vi "GetFrontPanel.vi"(8 "Error In":errorcluster, 11 "object in":refnum<class "FooterTriekselSoft.lvclass">) -> (0 "Error Out":errorcluster, 2 "FrontPanel":refnum<class "FrontPanelControl.lvclass">, 3 "object out":refnum<class "FooterTriekselSoft.lvclass">)   [LabVIEW 2021, in "FooterTriekselSoft.lvclass"]
uses:
  FooterTriekselSoft.lvclass
  .Externals/Library_UserInterface_FrontPanelControl/FrontPanelControl/FrontPanelControl.lvclass
  FooterGUI.vi
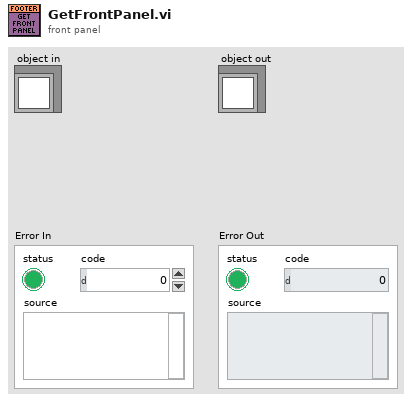
[diagram p1: front panel]
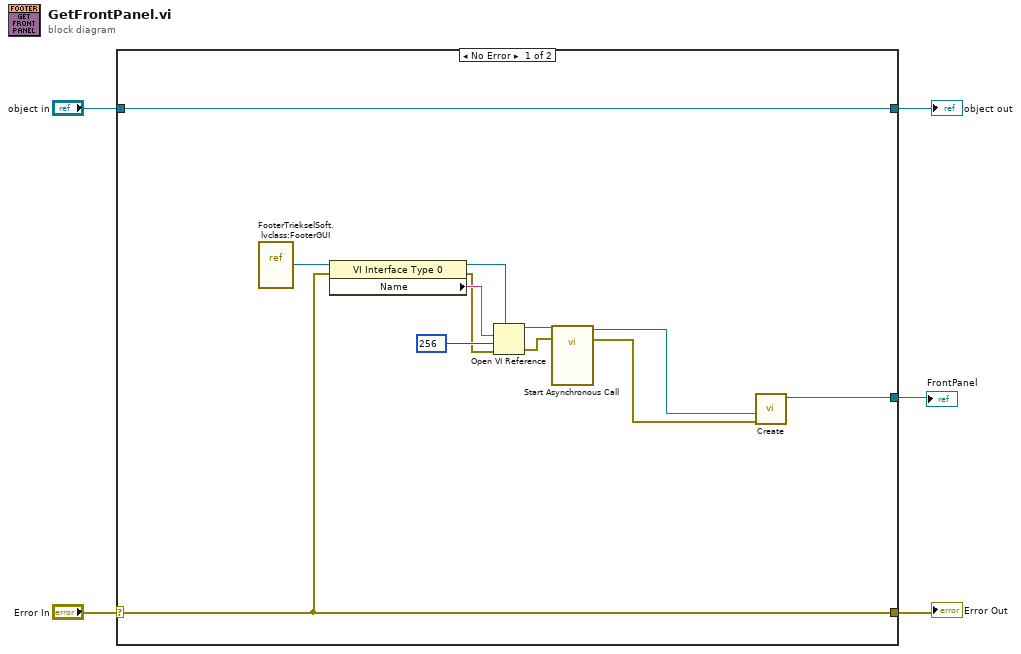
[diagram p0: block diagram]
diagram:
  n1 = case shown="No Error" "Error In" {
    selector: "Error In" -> [w7 w19]
    tunnel: [w7 w19] -> w4
    tunnel: [w17 w18] -> w2
    tunnel: "object in" -> [w17 w18]
    tunnel: [w6 _] -> w1
    frame No Error {
      n2 = vi-ref "FooterTriekselSoft.lvclass:FooterGUI.vi"() -> (w16:refnum<vi>)
      n3 = property class="VI Interface Type 0"(reference=w16, error in=w7) -> (reference out=w15:refnum<vi>, error out=w8:errorcluster, "Name"=w14:string)
      n4 = Open VI Reference(type specifier VI Refnum (for type only)=w15, vi path=w14, options=256, error in (no error)=w8) -> (vi reference=w12:refnum<vi>, error out=w11:errorcluster)  [unwired: 2 in]
      n5 = call-by-ref "Start Asynchronous Call"(reference=w12, error in=w11) -> (reference out=w10:refnum<vi>, error out=w9:errorcluster)  [unwired: 12 in]
      n6 = call "Create.vi"("ErrorIn"=w9, "VIRef"=w10) -> ("ObjectOut"=w6:refnum<class "FrontPanelControl.lvclass">)  [unwired: 8 in, 1 out]
    }
    frame Error {
    }
  }
  "Error Out" <- w4
  "object out" <- w2
  "FrontPanel" <- w1
